vi "IT8800-Read.vi"(8 "error in":errorcluster, 10 "byte count":u32, 11 "IT8800 Setting In In":T1={"VISA Resource Name"="", "Baud Rate"=19200, "Stop Bits"=20, "Wait For Read(ms)"=0, "Interface Type"=enum."VXI", "Limits"=[]} {"Stop Bits" items=["1.0"=10, "2.0"=20]; "Baud Rate" items=["2400"=2400, "4800"=4800, "9600"=9600, "19200"=19200]}) -> (0 "error out":errorcluster, 2 "Response":string, 3 "IT8800 Setting In Out":T1={"VISA Resource Name"="", "Baud Rate"=19200, "Stop Bits"=20, "Wait For Read(ms)"=0, "Interface Type"=enum."VXI", "Limits"=[]} {"Stop Bits" items=["1.0"=10, "2.0"=20]; "Baud Rate" items=["2400"=2400, "4800"=4800, "9600"=9600, "19200"=19200]})   [LabVIEW 2018]
uses:
  Data Def/IT8800-Setting.ctl
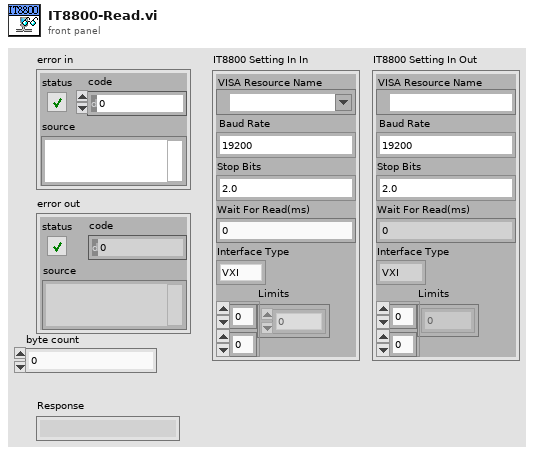
[diagram p1: front panel]
types:
  T1 = typedef "IT8800-Setting.ctl" = cluster{"VISA Resource Name":refnum<visa-resource-name>, "Baud Rate":u32, "Stop Bits":u16, "Wait For Read(ms)":u32, "Interface Type":enum16{"Unknow", "GPIB", "VXI", "GPIB-VXI", "Serial", "PXI", "TCPIP", "USB", "FireWire"}, "Limits":dbl[][]}
  T2 = enum16{"Unknow", "GPIB", "VXI", "GPIB-VXI", "Serial", "PXI", "TCPIP", "USB", "FireWire"}
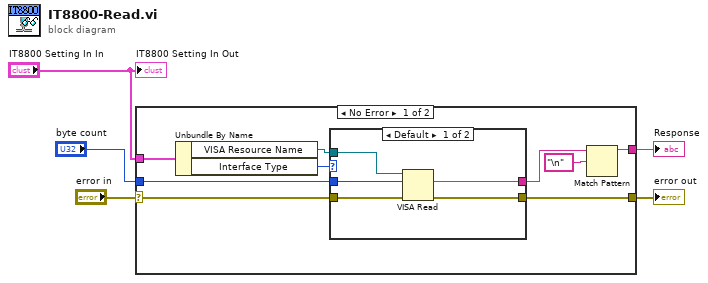
[diagram p0: block diagram]
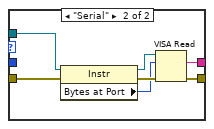
[diagram p2: hidden frame]
diagram:
  n1 = case shown="No Error" "error in" {
    selector: "error in" -> [w9 w27]
    tunnel: [w14 w27] -> w5
    tunnel: [w11 _] -> w4
    tunnel: "IT8800 Setting In In" -> [w10 _]
    tunnel: "byte count" -> [w6 _]
    frame No Error {
      n2 = Unbundle By Name(w10) -> ("VISA Resource Name"=w7:refnum<visa-resource-name>, "Interface Type"=w8:T2)
      n3 = case shown="Default" w8 {
        tunnel: w9 -> [w16 w20]
        tunnel: w7 -> [w19 w26]
        tunnel: [w18 w22] -> w13
        tunnel: [w17 w21] -> w14
        tunnel: w6 -> [w15 _]
        frame Default {
          n4 = VISA Read(VISA resource name=w19, byte count=w15, error in (no error)=w16) -> (read buffer=w18:string, error out=w17:errorcluster)  [unwired: 2 out]
        }
        frame "Serial" {
          n5 = property class="Instr"(reference=w26, error in=w20) -> (reference out=w25:refnum<visa-resource-name>, error out=w24:errorcluster, "Bytes at Port"=w23:u32)
          n6 = VISA Read(VISA resource name=w25, byte count=w23, error in (no error)=w24) -> (read buffer=w22:string, error out=w21:errorcluster)  [unwired: 2 out]
        }
      }
      n7 = Match Pattern(string=w13, regular expression="\n") -> (before substring=w11:string)  [unwired: 1 in, 3 out]
    }
    frame Error {
    }
  }
  "error out" <- w5
  "Response" <- w4
  "IT8800 Setting In Out" <- "IT8800 Setting In In"
